vi "Instr_InitObject.vi"(8 "error in (no error)":errorcluster, 9 "Instrument Configuration":variant, 10 "Instrument address":refnum<visa-resource-name>, 11 "LCRControl in":refnum<class "LCRControl.lvclass">) -> (0 "error out":errorcluster, 3 "LCRControl out":refnum<class "LCRControl.lvclass">)   [LabVIEW 2018, in "LCRControl.lvclass"]
uses:
  LCRControl.lvclass
  InstrControl.lvclass
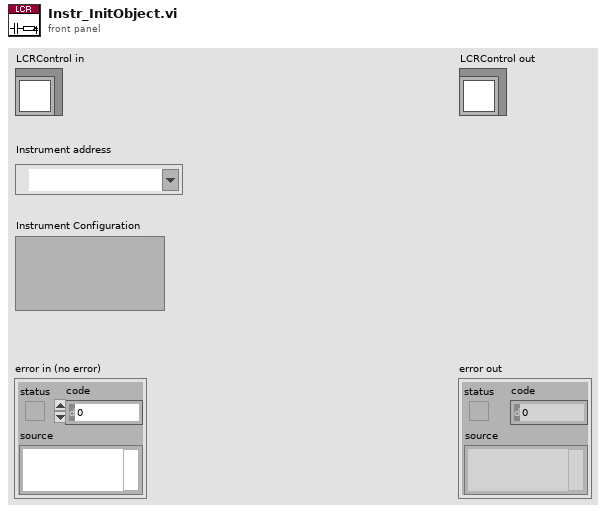
[diagram p1: front panel]
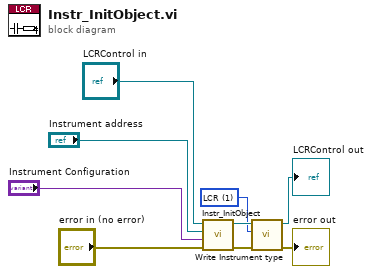
[diagram p0: block diagram]
diagram:
  w1 = u16 1 items=["Supply", "LCR", "Multimeter", "Switching"] ("Instrument type")
  n1 = call-parent "Instr_InitObject.vi"("error in (no error)"="error in (no error)", "Instrument Configuration"="Instrument Configuration", "Instrument address"="Instrument address", "InstrControl in"="LCRControl in") -> ("error out"=w5:errorcluster, "InstrControl out"=w7:refnum<class "LCRControl.lvclass">)  [unwired: 6 in]
  n2 = call-dynamic "Write Instrument type.vi"("error in (no error)"=w5, "Instrument type"=w1, "InstControl in"=w7) -> ("error out"=→"error out":errorcluster, "InstControl out"=→"LCRControl out":refnum<class "LCRControl.lvclass">)  [unwired: 7 in]
